vi "Cross Power (DBL).vi"(2 "Y":dbl[](array[numeric]), 3 "X":dbl[](array[numeric])) -> (0 "error":i32, 1 "Sxy":cdb[](array[numeric]))   [LabVIEW 2014, in "NI_AALPro.lvlib"]
doc: "Computes the cross power spectrum, <B>Sxy</B>, of the input signals <B>X</B> and <B>Y</B>. Wire data to the <B>X</B> input to determine the polymorphic instance to use or manually select the instance."
uses:
  NI_AALPro.lvlib
  lvanlys.dll
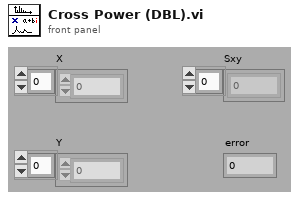
[diagram p1: front panel]
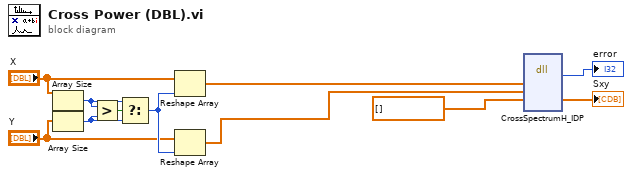
[diagram p0: block diagram]
diagram:
  n1 = Array Size(array="X") -> (size(s)=w9:i32)
  n2 = Array Size(array="Y") -> (size(s)=w8:i32)
  n3 = Greater?(x=w9, y=w8) -> (0:w10:bool)
  n4 = Select(t=w9, s=w10, f=w8) -> (s? t:f=w11:i32)
  n5 = Reshape Array("X", w11) -> (w4:dbl[])
  n6 = Reshape Array("Y", w11) -> (w5:dbl[])
  n7 = dll-call lib="C:/Program Files (x86)/National Instruments/LabVIEW 2014/resource/lvanlys.*" fn="CrossSpectrumH_IDP"("xH"=w4, "yH"=w5, "zH"=cdb[] [] ("Sxy")) -> ("return type"=→"error":i32, "zH"=→"Sxy":cdb[])  [unwired: 7 in, 2 out]
